vi "Setup.vi"(11 "Ex Queue Actor in":refnum<class "Ex Queue Actor.lvclass">) -> (3 "Ex Queue Actor out":refnum<class "Ex Queue Actor.lvclass">)   [LabVIEW 2021, in "Ex Queue Actor.lvlib" / "Ex Queue Actor.lvclass"]
uses:
  Ex Queue Actor.lvclass
  Ex Queue Actor.lvclass/Ex Queue Actor.ctl
  Actor/Queue Actor/Queue Actor.lvclass
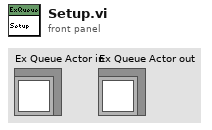
[diagram p1: front panel]
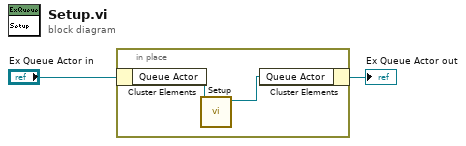
[diagram p0: block diagram]
diagram:
  n1 = in-place {
    n2 = in-place-cluster #1("Ex Queue Actor in") -> ("Queue Actor"=w4:refnum<class "Queue Actor.lvclass">)
    n3 = call-dynamic "Setup.vi"("Setup in"=w4) -> ("Setup out"=w3:refnum<class "Queue Actor.lvclass">)  [unwired: 10 in]
    n4 = in-place-cluster #1("Queue Actor"=w3) -> (→"Ex Queue Actor out":refnum<class "Ex Queue Actor.lvclass">)
  }
